vi "Create Hierarchy.vi"(8 "error in (no error)":errorcluster, 10 "Hierarchy":string[](array[string]), 11 "Config Manager in":refnum<class "Config Manager.lvclass">) -> (0 "error out":errorcluster, 2 "Leaf Element":refnum<class "Config Element.lvclass">, 3 "Config Manager out":refnum<class "Config Manager.lvclass">)   [LabVIEW 2023, in "CDM-Config.lvlib" / "Config Manager.lvclass"]
uses:
  Config Manager.lvclass
  Config Element/Config Element.lvclass
  Config Manager.lvclass/Config Manager.ctl
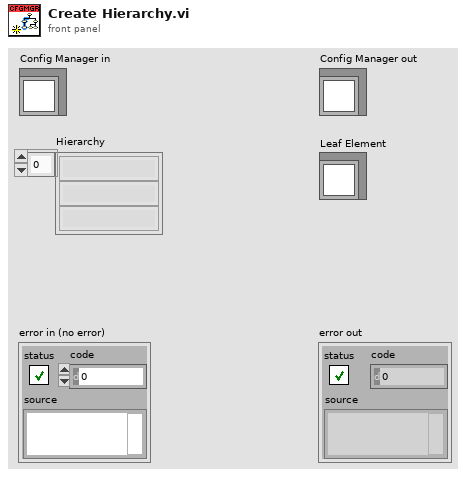
[diagram p1: front panel]
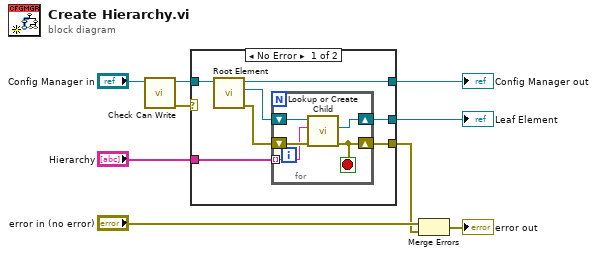
[diagram p0: block diagram]
diagram:
  n1 = call "Check Can Write.vi"("Config Manager in"="Config Manager in") -> ("error out"=w1:errorcluster, "Config Manager out"=w2:refnum<class "Config Manager.lvclass">)  [unwired: 9 in]
  n2 = case shown="No Error" w1 {
    selector: w1 -> [_ w22]
    tunnel: [w16 w23] -> w7
    tunnel: "Hierarchy" -> [w14 _]
    tunnel: [w13 _] -> w5
    tunnel: [w11 w22] -> w3
    tunnel: w2 -> [w10 w23]
    frame No Error {
      n3 = call "Root Element.vi"("Config Manager in"=w10) -> ("error out"=w12:errorcluster, "Root Element"=w15:refnum<class "Config Element.lvclass">, "Config Manager out"=w16:refnum<class "Config Manager.lvclass">)  [unwired: 8 in]
      n4 = for {
        tunnel: w14 -> [w19] mode=indexing
        shift-right: [w18] -> w13
        shift-left: w15 -> [w20]
        shift-right: [w17] -> w11
        shift-left: w12 -> [w21]
        stop <- w17 stop-if-true
        n5 = call "Lookup or Create Child.vi"("error in (no error)"=w21, "Name"=w19, "Config Element in"=w20) -> ("error out"=w17:errorcluster, "Child"=w18:refnum<class "Config Element.lvclass">)  [unwired: 5 in, 2 out]
      }
    }
    frame Error {
    }
  }
  "Config Manager out" <- w7
  "Leaf Element" <- w5
  n6 = Merge Errors("error in (no error)", w3) -> (→"error out":errorcluster)
